vi "myRIO v1.0 ISR Agent.vi"(7 "Run?":bool=TRUE, 8 "error in (no error)":errorcluster) -> (0 "error out":errorcluster)   [LabVIEW 2021]
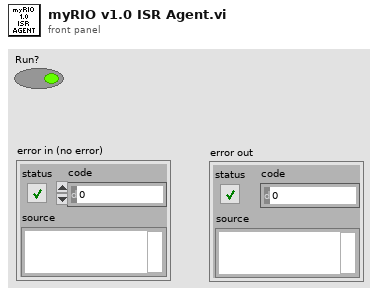
[diagram p1: front panel]
types:
  T1 = enum32{"Bad", "Idle", "Run top level", "Running"}
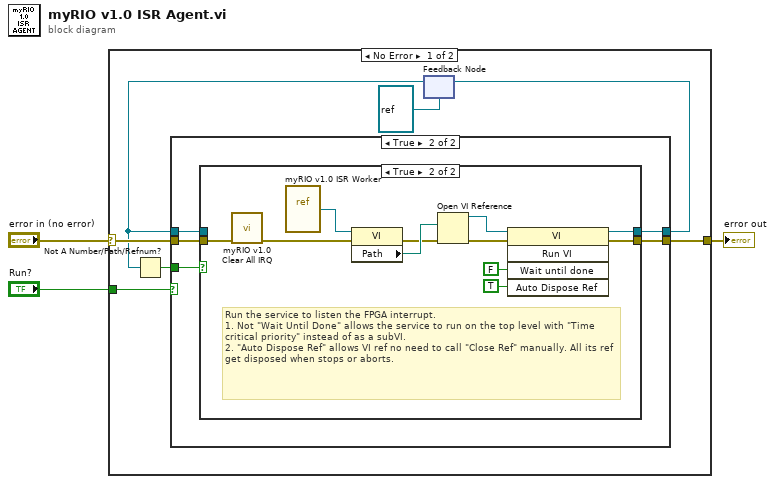
[diagram p0: block diagram]
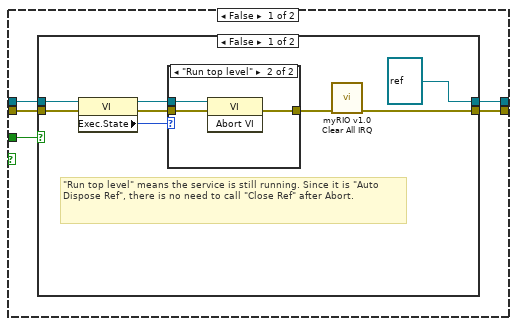
[diagram p2: hidden frame]
diagram:
  n1 = case shown="No Error" "error in (no error)" {
    selector: "error in (no error)" -> [w6 w48]
    tunnel: [w8 w48] -> w3
    tunnel: "Run?" -> [w7 _]
    frame No Error {
      n2 = feedback #1(refnum<vi> refnum) -> (w5:refnum<vi>)
      n3 = Not A Number/Path/Refnum?(number/path/refnum=w5) -> (NaN/Path/Refnum?=w4:bool)
      n4 = case shown="True" w7 {
        tunnel: [w15 w32] -> w10
        tunnel: w5 -> [w13 w34]
        tunnel: [w14 w31] -> w8
        tunnel: w6 -> [w12 w33]
        tunnel: w4 -> [w11 w30]
        frame False {
          n5 = case shown="False" w11 {
            tunnel: [refnum<vi> refnum w29] -> w15
            tunnel: [w21 w28] -> w14
            tunnel: w13 -> [w20 w29]
            tunnel: w12 -> [w19 w28]
            frame False {
              # "\"Run top level\" means the service is still running. Since it is \"Auto Dispose Ref\", there is no need to call \"Close Ref\" after Abort."
              n6 = property class="VI"(reference=w20, error in=w19) -> (reference out=w17:refnum<vi>, error out=w16:errorcluster, "Exec.State"=w18:T1)
              n7 = case shown="\"Run top level\"" w18 {
                tunnel: [w24 w27] -> w22
                tunnel: w17 -> [_ w26]
                tunnel: w16 -> [w24 w25]
                frame Default {
                }
                frame "Run top level" {
                  n8 = invoke class="VI" method="Abort VI"(reference=w26, error in=w25) -> (error out=w27:errorcluster)  [unwired: 1 in, 2 out]
                }
              }
              n9 = call <vilib>:"myRIO v1.0 Clear All IRQ.vi"("error in (no error)"=w22) -> ("error out"=w21:errorcluster)  [unwired: 10 in]
            }
            frame True {
              # "Service is stopped. Do nothing."
            }
          }
        }
        frame True {
          n10 = case shown="True" w30 {
            tunnel: w34 -> [w36 _]
            tunnel: w33 -> [w35 w44]
            tunnel: [w36 w39] -> w32
            tunnel: [w35 w37] -> w31
            frame False {
              # "Service is running. Do nothing."
            }
            frame True {
              # "Run the service to listen the FPGA interrupt.\n1. Not \"Wait Until Done\" allows the service to run on the top level with \"Time critical priority\" instead of as a subVI.\n2. \"Auto Dispose Ref\" allows VI ref no need to call \"Close Ref\" manually. All its ref get disposed when stops or aborts."
              n11 = call <vilib>:"myRIO v1.0 Clear All IRQ.vi"("error in (no error)"=w44) -> ("error out"=w43:errorcluster)  [unwired: 10 in]
              n12 = vi-ref <vilib>:"myRIO v1.0 ISR Worker.vi"() -> (w45:refnum<vi>)
              n13 = property class="VI"(reference=w45, error in=w43) -> (error out=w46:errorcluster, "Path"=w47:path)  [unwired: 1 out]
              n14 = Open VI Reference(vi path=w47, error in (no error)=w46) -> (vi reference=w40:refnum<vi>, error out=w38:errorcluster)  [unwired: 4 in]
              n15 = invoke class="VI" method="Run VI"(reference=w40, error in=w38, "Wait until done"=FALSE ("Wait Until Done"), "Auto Dispose Ref"=TRUE ("Auto Dispose Reference")) -> (reference out=w39:refnum<vi>, error out=w37:errorcluster)  [unwired: 1 in, 3 out]
            }
          }
        }
      }
      n16 = feedback-in #1(w10) -> ()
    }
    frame Error {
    }
  }
  "error out" <- w3
